vi "Getenet.vi"(8 "error in (no error)":errorcluster, 11 "OneOfTemplate in":refnum<class "nixnet_grpc_FrameBufferRequest_frame.lvclass">) -> (0 "error out":errorcluster, 2 "Get_Val":T1, 3 "OneOfTemplate out":refnum<class "nixnet_grpc_FrameBufferRequest_frame.lvclass">)   [LabVIEW 2019, in "grpc-xnet_client.lvlib" / "nixnet_grpc_FrameBufferRequest_frame.lvclass"]
uses:
  nixnet_grpc_FrameBufferRequest_frame.lvclass
  nixnet_grpc_EnetFrameRequest.ctl
  nixnet_grpc_EnetFrameRequest_type_enum/nixnet_grpc_EnetFrameRequest_type_enum.lvclass
  nixnet_grpc_EnetFlags.ctl
  nixnet_grpc_FrameBufferRequest_frame.lvclass/nixnet_grpc_FrameBufferRequest_frame.ctl
  grpc-xnet_client.lvlib
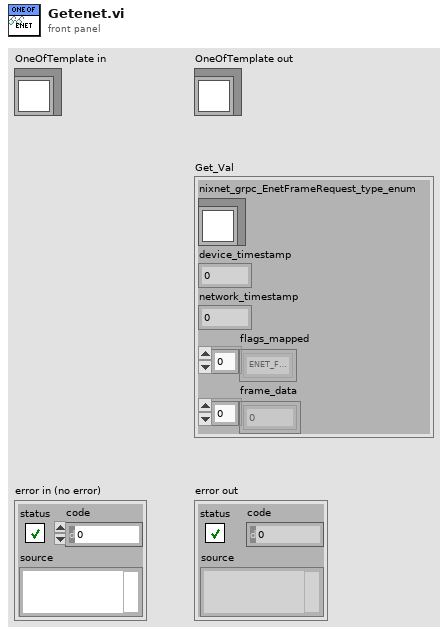
[diagram p1: front panel]
types:
  T1 = typedef "grpc-xnet_client.lvlib/nixnet_grpc_EnetFrameRequest.ctl" = cluster{"nixnet_grpc_EnetFrameRequest_type_enum":refnum<class "nixnet_grpc_EnetFrameRequest_type_enum.lvclass">, "device_timestamp":u64, "network_timestamp":u64, "flags_mapped":T2[], "frame_data":u8[]}
  T2 = typedef "grpc-xnet_client.lvlib/nixnet_grpc_EnetFlags.ctl" = enum32{"ENET_FLAGS_UNSPECIFIED", "ENET_FLAGS_TRANSMIT", "ENET_FLAGS_RECEIVE", "ENET_FLAGS_NETWORK_SYNCED", "ENET_FLAGS_ERROR"}
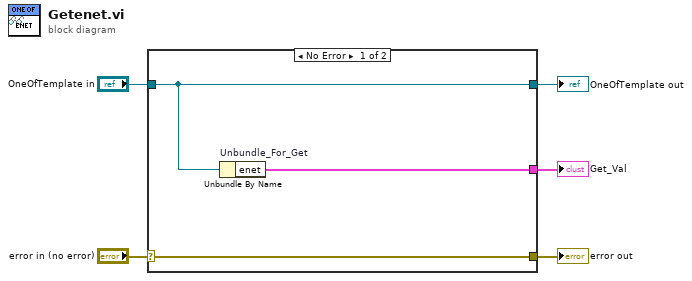
[diagram p0: block diagram]
diagram:
  n1 = case shown="No Error" "error in (no error)" {
    selector: "error in (no error)" -> [w8 w9]
    tunnel: [w8 w9] -> w4
    tunnel: [w7 w10] -> w2
    tunnel: "OneOfTemplate in" -> [w7 w10]
    tunnel: [w6 _] -> w1
    frame No Error {
      n2 = Unbundle By Name "Unbundle_For_Get"(w7) -> ("enet"=w6:T1)
    }
    frame Error {
    }
  }
  "error out" <- w4
  "OneOfTemplate out" <- w2
  "Get_Val" <- w1
